vi "Test Basic.vi"(8 "error in (no error)":errorcluster) -> (0 "error out":errorcluster)   [LabVIEW 2020]
uses:
  Source/Protobuf RAW/uint32/uint32.lvclass/uint32.ctl
  Source/Protobuf RAW/bool/bool.lvclass/bool.ctl
  Source/Protobuf RAW/sint64/sint64.lvclass/sint64.ctl
  Source/Protobuf RAW/uint64/uint64.lvclass/uint64.ctl
  Source/Protobuf RAW/sint32/sint32.lvclass/sint32.ctl
  Source/Protobuf RAW/int64/int64.lvclass/int64.ctl
  Source/Protobuf RAW/int32/int32.lvclass/int32.ctl
  Source/Protobuf RAW/int32/Write Value.vi
  Source/Protobuf RAW/int64/Write Value.vi
  Source/Protobuf RAW/sint32/Write Value.vi
  Source/Protobuf RAW/bool/Write Value.vi
  Source/Protobuf RAW/uint64/Write Value.vi
  Source/Protobuf RAW/sint64/Write Value.vi
  Source/Protobuf RAW/uint32/Write Value.vi
  Source/Protobuf RAW/uint32/uint32.lvclass
  Source/Protobuf RAW/bool/bool.lvclass
  Source/Protobuf RAW/sint64/sint64.lvclass
  Source/Protobuf RAW/uint64/uint64.lvclass
  Source/Protobuf RAW/sint32/sint32.lvclass
  Source/Protobuf RAW/int64/int64.lvclass
  Source/Protobuf RAW/int32/int32.lvclass
  Source/Protobuf RAW.lvlib
  <vilib>/addons/_JKI Toolkits/Caraya/classes/Assert/Assert.lvclass
  <vilib>/addons/_JKI Toolkits/Caraya/classes/Test/Test.lvclass
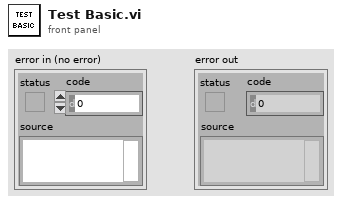
[diagram p1: front panel]
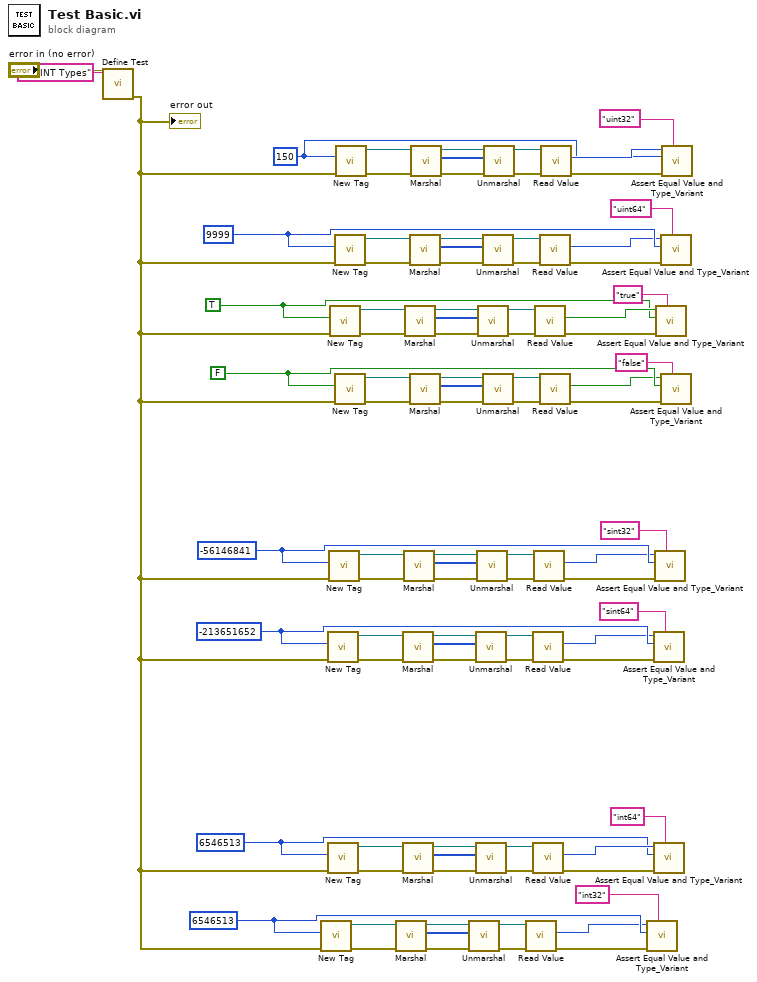
[diagram p0: block diagram]
diagram:
  w12 = FALSE
  w23 = i64 -213651652
  w34 = 6546513
  w39 = i64 6546513
  w56 = -56146841
  w61 = TRUE
  w78 = u64 9999
  w82 = u32 150
  n1 = call <vilib>:"Define Test.vi"("error in (no error)"="error in (no error)", "Label (VI Title)"="VarINT Types") -> ("error out"=w3:errorcluster)  [unwired: 9 in]
  "error out" <- w3
  n2 = call-poly "New Tag.vi"("error in (no error)"=w3, "Value"=w34) -> ("error out"=w30:errorcluster, "int32 out"=w27:refnum<class "int32.lvclass">)  [unwired: 8 in]
  n3 = call-poly "New Tag.vi"("error in (no error)"=w3, "Value"=w23) -> ("error out"=w19:errorcluster, "int32 out"=w16:refnum<class "sint64.lvclass">)  [unwired: 8 in]
  n4 = call-poly "New Tag.vi"("error in (no error)"=w3, "Value"=w39) -> ("error out"=w43:errorcluster, "int32 out"=w46:refnum<class "int64.lvclass">)  [unwired: 8 in]
  n5 = call-poly "New Tag.vi"("error in (no error)"=w3, "Value"=w56) -> ("error out"=w52:errorcluster, "int32 out"=w49:refnum<class "sint32.lvclass">)  [unwired: 8 in]
  n6 = call-poly "New Tag.vi"("error in (no error)"=w3, "Value"=w61) -> ("error out"=w65:errorcluster, "int32 out"=w68:refnum<class "bool.lvclass">)  [unwired: 8 in]
  n7 = call-poly "New Tag.vi"("error in (no error)"=w3, "Value"=w78) -> ("error out"=w74:errorcluster, "int32 out"=w71:refnum<class "uint64.lvclass">)  [unwired: 8 in]
  n8 = call-poly "New Tag.vi"("error in (no error)"=w3, "Value"=w12) -> ("error out"=w8:errorcluster, "int32 out"=w5:refnum<class "bool.lvclass">)  [unwired: 8 in]
  n9 = call-poly "New Tag.vi"("error in (no error)"=w3, "Value"=w82) -> ("error out"=w87:errorcluster, "int32 out"=w90:refnum<class "uint32.lvclass">)  [unwired: 8 in]
  n10 = call-dynamic "Marshal.vi"("error in (no error)"=w30, "int32 in"=w27) -> ("error out"=w31:errorcluster, "Buffer"=w28:u8[], "int32 out"=w26:refnum<class "int32.lvclass">)  [unwired: 7 in]
  n11 = call-dynamic "Marshal.vi"("error in (no error)"=w19, "int32 in"=w16) -> ("error out"=w20:errorcluster, "Buffer"=w17:u8[], "int32 out"=w15:refnum<class "sint64.lvclass">)  [unwired: 7 in]
  n12 = call-dynamic "Marshal.vi"("error in (no error)"=w43, "int32 in"=w46) -> ("error out"=w42:errorcluster, "Buffer"=w45:u8[], "int32 out"=w47:refnum<class "int64.lvclass">)  [unwired: 7 in]
  n13 = call-dynamic "Marshal.vi"("error in (no error)"=w52, "int32 in"=w49) -> ("error out"=w53:errorcluster, "Buffer"=w50:u8[], "int32 out"=w48:refnum<class "sint32.lvclass">)  [unwired: 7 in]
  n14 = call-dynamic "Marshal.vi"("error in (no error)"=w65, "int32 in"=w68) -> ("error out"=w64:errorcluster, "Buffer"=w67:u8[], "int32 out"=w69:refnum<class "bool.lvclass">)  [unwired: 7 in]
  n15 = call-dynamic "Marshal.vi"("error in (no error)"=w74, "int32 in"=w71) -> ("error out"=w75:errorcluster, "Buffer"=w72:u8[], "int32 out"=w70:refnum<class "uint64.lvclass">)  [unwired: 7 in]
  n16 = call-dynamic "Marshal.vi"("error in (no error)"=w8, "int32 in"=w5) -> ("error out"=w9:errorcluster, "Buffer"=w6:u8[], "int32 out"=w4:refnum<class "bool.lvclass">)  [unwired: 7 in]
  n17 = call-dynamic "Marshal.vi"("error in (no error)"=w87, "int32 in"=w90) -> ("error out"=w86:errorcluster, "Buffer"=w89:u8[], "int32 out"=w91:refnum<class "uint32.lvclass">)  [unwired: 7 in]
  n18 = call-dynamic "Unmarshal.vi"("error in (no error)"=w31, "Buffer"=w28, "int32 in"=w26) -> ("error out"=w32:errorcluster, "int32 out"=w29:refnum<class "int32.lvclass">)  [unwired: 6 in, 1 out]
  n19 = call-dynamic "Unmarshal.vi"("error in (no error)"=w20, "Buffer"=w17, "int32 in"=w15) -> ("error out"=w21:errorcluster, "int32 out"=w18:refnum<class "sint64.lvclass">)  [unwired: 6 in, 1 out]
  n20 = call-dynamic "Unmarshal.vi"("error in (no error)"=w42, "Buffer"=w45, "int32 in"=w47) -> ("error out"=w41:errorcluster, "int32 out"=w44:refnum<class "int64.lvclass">)  [unwired: 6 in, 1 out]
  n21 = call-dynamic "Unmarshal.vi"("error in (no error)"=w53, "Buffer"=w50, "int32 in"=w48) -> ("error out"=w54:errorcluster, "int32 out"=w51:refnum<class "sint32.lvclass">)  [unwired: 6 in, 1 out]
  n22 = call-dynamic "Unmarshal.vi"("error in (no error)"=w64, "Buffer"=w67, "int32 in"=w69) -> ("error out"=w63:errorcluster, "int32 out"=w66:refnum<class "bool.lvclass">)  [unwired: 6 in, 1 out]
  n23 = call-dynamic "Unmarshal.vi"("error in (no error)"=w75, "Buffer"=w72, "int32 in"=w70) -> ("error out"=w76:errorcluster, "int32 out"=w73:refnum<class "uint64.lvclass">)  [unwired: 6 in, 1 out]
  n24 = call-dynamic "Unmarshal.vi"("error in (no error)"=w9, "Buffer"=w6, "int32 in"=w4) -> ("error out"=w10:errorcluster, "int32 out"=w7:refnum<class "bool.lvclass">)  [unwired: 6 in, 1 out]
  n25 = call-dynamic "Unmarshal.vi"("error in (no error)"=w86, "Buffer"=w89, "int32 in"=w91) -> ("error out"=w85:errorcluster, "int32 out"=w88:refnum<class "uint32.lvclass">)  [unwired: 6 in, 1 out]
  n26 = call "Read Value.vi"("error in (no error)"=w32, "int32 in"=w29) -> ("error out"=w35:errorcluster, "Value"=w33:i32)  [unwired: 7 in, 1 out]
  n27 = call "Read Value.vi"("error in (no error)"=w21, "int32 in"=w18) -> ("error out"=w24:errorcluster, "Value"=w22:i64)  [unwired: 7 in, 1 out]
  n28 = call "Read Value.vi"("error in (no error)"=w41, "int32 in"=w44) -> ("error out"=w38:errorcluster, "Value"=w40:i64)  [unwired: 7 in, 1 out]
  n29 = call "Read Value.vi"("error in (no error)"=w54, "int32 in"=w51) -> ("error out"=w57:errorcluster, "Value"=w55:i32)  [unwired: 7 in, 1 out]
  n30 = call "Read Value.vi"("error in (no error)"=w63, "int32 in"=w66) -> ("error out"=w60:errorcluster, "Value"=w62:bool)  [unwired: 7 in, 1 out]
  n31 = call "Read Value.vi"("error in (no error)"=w76, "int32 in"=w73) -> ("error out"=w79:errorcluster, "Value"=w77:u64)  [unwired: 7 in, 1 out]
  n32 = call "Read Value.vi"("error in (no error)"=w10, "int32 in"=w7) -> ("error out"=w13:errorcluster, "Value"=w11:bool)  [unwired: 7 in, 1 out]
  n33 = call "Read Value.vi"("error in (no error)"=w85, "int32 in"=w88) -> ("error out"=w81:errorcluster, "Value"=w83:u32)  [unwired: 7 in, 1 out]
  n34 = call <vilib>:"Assert Equal Value and Type_Variant.vi"("Label"="int32", "error in (no error)"=w35, "Y"=w34, "X"=w33) -> ()  [unwired: 7 in, 1 out]
  n35 = call <vilib>:"Assert Equal Value and Type_Variant.vi"("Label"="sint64", "error in (no error)"=w24, "Y"=w23, "X"=w22) -> ()  [unwired: 7 in, 1 out]
  n36 = call <vilib>:"Assert Equal Value and Type_Variant.vi"("Label"="int64", "error in (no error)"=w38, "Y"=w39, "X"=w40) -> ()  [unwired: 7 in, 1 out]
  n37 = call <vilib>:"Assert Equal Value and Type_Variant.vi"("Label"="sint32", "error in (no error)"=w57, "Y"=w56, "X"=w55) -> ()  [unwired: 7 in, 1 out]
  n38 = call <vilib>:"Assert Equal Value and Type_Variant.vi"("Label"="true", "error in (no error)"=w60, "Y"=w61, "X"=w62) -> ()  [unwired: 7 in, 1 out]
  n39 = call <vilib>:"Assert Equal Value and Type_Variant.vi"("Label"="uint64", "error in (no error)"=w79, "Y"=w78, "X"=w77) -> ()  [unwired: 7 in, 1 out]
  n40 = call <vilib>:"Assert Equal Value and Type_Variant.vi"("Label"="false", "error in (no error)"=w13, "Y"=w12, "X"=w11) -> ()  [unwired: 7 in, 1 out]
  n41 = call <vilib>:"Assert Equal Value and Type_Variant.vi"("Label"="uint32", "error in (no error)"=w81, "Y"=w82, "X"=w83) -> ()  [unwired: 7 in, 1 out]
